vi "Teardown.vi"(7 "Is Sync":bool) -> (2 "Msg":refnum<class "Msg.lvclass">)   [LabVIEW 2020, in "jettl.lvlib" / "Teardown Msg.lvlib"]
uses:
  Teardown Msg.lvlib
  Teardown Msg/Teardown Msg.lvclass
  Msg/Msg.lvclass
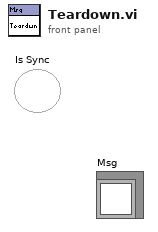
[diagram p1: front panel]
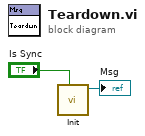
[diagram p0: block diagram]
diagram:
  n1 = call "Init.vi"("Is Sync"="Is Sync") -> ("Teardown Msg out"=→"Msg":refnum<class "Teardown Msg.lvclass">)  [unwired: 10 in]
